vi "Label Translate.vi"(11 "String In":string) -> (0 "Test Result":bool, 1 "Label OK":bool, 2 "SN or ID":i32, 3 "DTandShift":string)   [LabVIEW 2018]
panel:
  # "OK\nE180639 190718D 000002"
  # "NG\nE180639 190718D 1135 1 NGxxx 484"
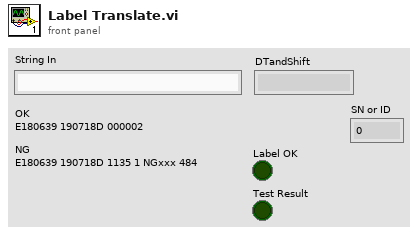
[diagram p1: front panel]
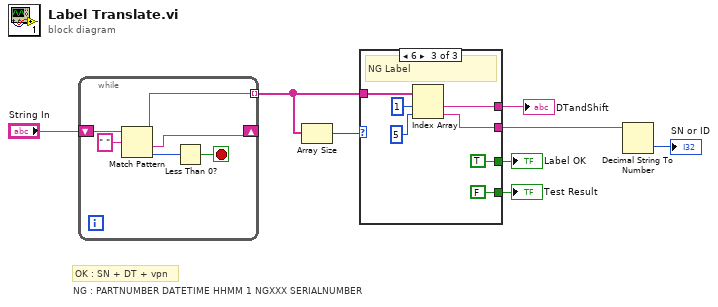
[diagram p0: block diagram]
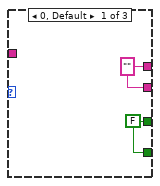
[diagram p2: hidden frame]
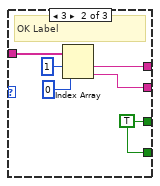
[diagram p3: hidden frame]
diagram:
  # "NG : PARTNUMBER DATETIME HHMM 1 NGXXX SERIALNUMBER"
  # "OK : SN + DT + vpn"
  n1 = while {
    shift-right: [w11] -> _
    shift-left: "String In" -> [w14]
    tunnel: [w12] -> w7 mode=indexing
    stop <- w9 stop-if-true
    n2 = Match Pattern(string=w14, regular expression=" ") -> (before substring=w12:string, after substring=w11:string, offset past match=w10:i32)  [unwired: 1 in, 1 out]
    n3 = Less Than 0?(x=w10) -> (x < 0?=w9:bool)
  }
  n4 = Array Size(array=w7) -> (size(s)=w6:i32)
  n5 = case shown="6" w6 {
    tunnel: w7 -> [_ w21 w28]
    tunnel: [w16 w20 w26] -> w5
    tunnel: [w16 w18 w25] -> w2
    tunnel: [w15 w17 TRUE] -> w4
    tunnel: [w15 w17 FALSE] -> w3
    frame 0, Default {
      w15 = FALSE
      w16 = "" ("String In")
    }
    frame 3 {
      w17 = TRUE
      # "OK Label"
      n6 = Index Array(array=w21, index #1=1 ("index"), index #2=0 ("index")) -> (element #1=w20:string, element #2=w18:string)
    }
    frame 6 {
      # "NG Label"
      n7 = Index Array(array=w28, index #1=1 ("index"), index #2=5 ("index")) -> (element #1=w26:string, element #2=w25:string)
    }
  }
  "DTandShift" <- w5
  "Label OK" <- w4
  "Test Result" <- w3
  n8 = Decimal String To Number(string=w2) -> (number=→"SN or ID":i32)  [unwired: 2 in, 1 out]
